vi "GMLAN ProgrammingMode.vi"(8 "error in (no error)":errorcluster, 10 "subFunction":T1=1 items=["requestProgrammingMode"=1, "requestProgrammingMode_HighSpeed"=2, "enableProgrammingMode"=3], 11 "diag ref in":T2) -> (0 "error out":errorcluster, 1 "success?":bool, 3 "diag ref out":T2)   [LabVIEW 2015, in "GMLAN.lvlib"]
uses:
  GMLAN.lvlib
  <vilib>/Automotive Diagnostic Command Set/Diagnostic Transport.llb/Diag Reference.ctl
  <vilib>/Automotive Diagnostic Command Set/Diagnostic Transport.llb/Transport Protocol Selector.ctl
  <vilib>/Automotive Diagnostic Command Set/Diagnostic Transport.llb/Diag CAN Frame Log.ctl
  _SubVIs/ProgrammingMode_SubFunction.ctl
  <vilib>/Automotive Diagnostic Command Set/Diagnostic Transport.llb/Apply Diagnostic Error.vi
  <vilib>/Automotive Diagnostic Command Set/Diagnostic Transport.llb/Diagnostic Response Recv.vi
  <vilib>/Automotive Diagnostic Command Set/Diagnostic Transport.llb/Diagnostic Service Send.vi
  <vilib>/Automotive Diagnostic Command Set/Diagnostic Transport.llb/Diag Globals.vi
  <vilib>/addons/Automotive Diagnostic Command Set/NI_Automotive Diagnostic Command Set.lvlib
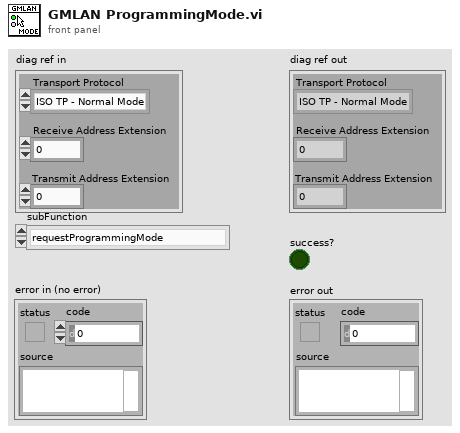
[diagram p1: front panel]
types:
  T1 = typedef "GMLAN.lvlib/ProgrammingMode_SubFunction.ctl" = u8
  T2 = typedef "NI_Automotive Diagnostic Command Set.lvlib/Diag Reference.ctl" = cluster{"Diag CAN Handle":u32, "Transport Protocol":T3, "Receive Address Extension":u8, "Transmit Address Extension":u8, "Receive CAN Id":u32, "Transmit CAN Id":u32, "Diag CAN Queue":refnum<queue>, "Log Frames ?":bool, "My TP Address":u8, "Other TP Address":u8, "T1":u16, "T2":u16, "T3":u16, "T4":u16, "Tx SN":u8, "Block Size":u8, "Rx SN":u8, "VW TP Initialized?":bool, "Tx block no":u8, "baud rate":u32, "Interface":string, "Channel Diag CAN Handle":u32, "UDP Connection ID":refnum<k16>, "TCP Connection ID":refnum<k5>, "Target IP Addr":u32, "Source Address":u16, "Target Address":u16, "Send Header NACK?":bool, "DLL Handle":u32, "NAD":u8, "Time Stamp read first":dbl, "Time Stamp read last":dbl, "Time Stamp write first":dbl, "Time Stamp write last":dbl, "Time Stamp write":dbl, "Time Stamp read":dbl}
  T3 = typedef "NI_Automotive Diagnostic Command Set.lvlib/Transport Protocol Selector.ctl" = enum16{"ISO TP - Normal Mode", "ISO TP - Mixed Mode", "VW TP 2.0", "Diagnostics on IP", "ISO TP LIN"}
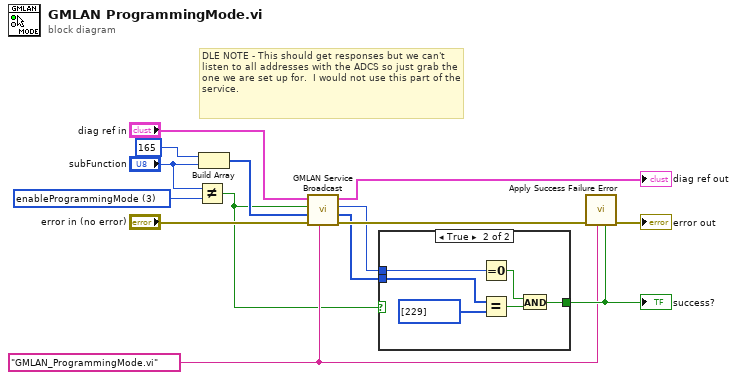
[diagram p0: block diagram]
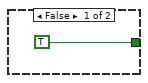
[diagram p2: hidden frame]
diagram:
  w2 = T1 3 items=["requestProgrammingMode"=1, "requestProgrammingMode_HighSpeed"=2, "enableProgrammingMode"=3] ("y")
  w5 = "GMLAN_ProgrammingMode.vi" ("error source")
  # "DLE NOTE - This should get responses but we can't listen to all addresses with the ADCS so just grab the one we are set up for.  I would not use this part of the service."
  n1 = Not Equal?(x="subFunction", y=w2) -> (x != y?=w1:bool)
  n2 = Build Array(u8 165, "subFunction") -> (w10:T1[])
  n3 = call "GMLAN Service Broadcast.vi"("error source"=w5, "error in (no error)"="error in (no error)", "data in"=w10, "require response?"=w1, "diag ref in"="diag ref in") -> ("error out"=w7:errorcluster, "data out"=w4:u8[], "error code"=w6:u8, "diag ref out"=→"diag ref out":T2)  [unwired: 3 in]
  n4 = case shown="True" w1 {
    tunnel: [TRUE w18] -> w9
    tunnel: w6 -> [_ w17]
    tunnel: w4 -> [_ w16]
    frame False {
    }
    frame True {
      n5 = Equal To 0?(x=w17) -> (x = 0?=w19:bool)
      n6 = Equal?(x=w16, y=u8[] [229]) -> (x = y?=w20:bool)
      n7 = And(x=w19, y=w20) -> (x .and. y?=w18:bool)
    }
  }
  "success?" <- w9
  n8 = call <vilib>:"Apply Success Failure Error.vi"("success code"=w9, "error source"=w5, "error in (no error)"=w7) -> ("error out"=→"error out":errorcluster)  [unwired: 8 out]
